vi "3D ANOVA.vi"(0 "X":dbl[](array[numeric]) format="%0.4f", 1 "Levels":T2={"Level A"=2, "Level B"=2, "Level C"=2} {"Level C" format="%0.0f"; "Level B" format="%0.0f"; "Level A" format="%0.0f"}, 2 "Index A":i32[](array[numeric]), 3 "Index B":i32[](array[numeric]) format="%0.0f", 4 "observations per cell":i32=2 format="%0.0f", 5 "Index C":i32[](array[numeric]) format="%0.0f") -> (6 "Info":dbl[][](array[numeric]) format="%0.4f", 7 "Significance":T1 {"sig ABC" format="%0.4f"; "sig BC" format="%0.4f"; "sig AC" format="%0.4f"; "sig AB" format="%0.4f"; "sig C" format="%0.4f"; "sig B" format="%0.4f"; "sig A" format="%0.4f"}, 8 "error":i32)   [LabVIEW 2020, in "NI_AALPro.lvlib"]
doc: "Takes an array of experimental observations made at various levels of three factors and performs a three-way analysis of variance."
uses:
  <vilib>/Analysis/NI_AALPro.lvlib
  <resource>/lvanlys.dll
panel:
  # "3D ANOVA"
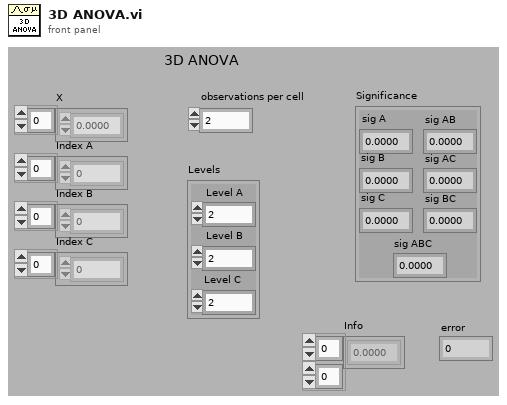
[diagram p1: front panel]
types:
  T1 = cluster{"sig A":dbl, "sig B":dbl, "sig C":dbl, "sig AB":dbl, "sig AC":dbl, "sig BC":dbl, "sig ABC":dbl}
  T2 = cluster{"Level A":i32, "Level B":i32, "Level C":i32}
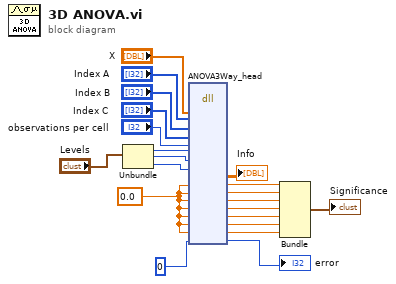
[diagram p0: block diagram]
diagram:
  w13 = 0.0
  n1 = Unbundle("Levels") -> ("Level A"=w16:i32, "Level B"=w15:i32, "Level C"=w14:i32)
  n2 = dll-call lib="e:/builds/penguin/labview/branches/2020/dev/dist/resource/lvanlys.*" fn="ANOVA3Way_head"("X"="X", "Index A"="Index A", "Index B"="Index B", "Index C"="Index C", "observations per cell"="observations per cell", "Level A"=w16, "Level B"=w15, "Level C"=w14, w13, w13, w13, w13, w13, w13, w13, 0) -> ("Info"=→"Info":dbl[][], w10:dbl, w9:dbl, w8:dbl, w7:dbl, w6:dbl, w5:dbl, w4:dbl, →"error":i32)  [unwired: 13 in, 2 out]
  n3 = Bundle(w10, w9, w8, w7, w6, w5, w4) -> (→"Significance":cluster{dbl, dbl, dbl, dbl, dbl, dbl, dbl})  [unwired: 1 in]
